vi "Test.vi"(11 "reference":refnum<k24>) -> (3 "Position X(mm)":dbl)   [LabVIEW 2020]
uses:
  F:/Labview_Control_SIC/Labview Kinesis/Thorlabs.MotionControl.Controls.dll
  Labview Kinesis/Thorlabs.MotionControl.Controls.dll
  F:/Labview_Control_SIC/Labview Kinesis/ThorLabs.MotionControl.KCube.DCServoCLI.dll
  Labview Kinesis/ThorLabs.MotionControl.KCube.DCServoCLI.dll
panel:
  in  "SerialNumberX":string="27004363"
  out "error out":errorcluster
  out "CreateDevice":bool
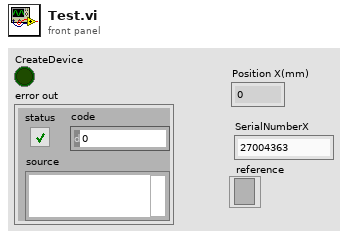
[diagram p1: front panel]
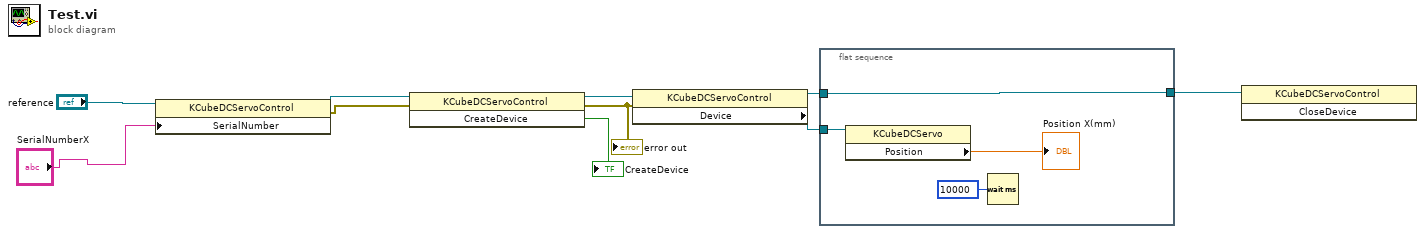
[diagram p0: block diagram]
diagram:
  n1 = property class="KCubeDCServoControl"(reference="reference", "SerialNumber"="SerialNumberX") -> (reference out=w10:refnum<k24>, error out=w8:errorcluster)  [unwired: 1 in]
  n2 = invoke class="KCubeDCServoControl" method="CreateDevice"(reference=w10, error in=w8) -> (reference out=w9:refnum<k24>, error out=w7:errorcluster, "CreateDevice"=→"CreateDevice":bool)  [unwired: 1 in]
  "error out" <- w7
  n3 = property class="KCubeDCServoControl"(reference=w9, error in=w7) -> (reference out=w5:refnum<k24>, "Device"=w6:refnum<k24>)  [unwired: 1 out]
  n4 = flat-sequence {
    tunnel: w6 -> [w14]
    tunnel: [w13] -> w4
    tunnel: w5 -> [w13]
    frame #0 {
      n5 = property class="KCubeDCServo"(reference=w14) -> ("Position"=→"Position X(mm)":dbl)  [unwired: 1 in, 2 out]
      n6 = Wait (ms)(milliseconds to wait=u32 10000) -> ()  [unwired: 1 out]
    }
  }
  n7 = invoke class="KCubeDCServoControl" method="CloseDevice"(reference=w4) -> ()  [unwired: 2 in, 3 out]
